vi "Stand Alone Init.vi"() -> (0 "error out":errorcluster, 1 "Engine Parent Editor Node":refnum<data-value>, 3 "Scan Engine Editor Node":refnum<data-value>)   [LabVIEW 2013, in "Scan Engine editor node.lvclass"]
uses:
  Scan Engine editor node.lvclass
  <vilib>/NI/Tag Bus Data Framework/Configuration Editor/Classes/Engine Parent/Engine Parent Editor Node.lvclass
  <vilib>/NI/Tag Bus/tag/tag descriptor.lvclass
  <vilib>/NI/Tag Bus/tag/Data Type.ctl
  module/configuration/Scan Engine configuration.lvclass
  <vilib>/NI/Module Execution Interface/Engine Configuration/engine configuration.lvclass
  <vilib>/NI/Tag Bus/tag/tag descriptor.lvclass/tag descriptor.ctl
  <vilib>/NI/Tag Bus/tag/write tag name.vi
  <vilib>/NI/Tag Bus/tag/write data type.vi
  <vilib>/NI/Tag Bus Data Framework/Configuration Editor/Classes/Engine Parent/write engine configuration.vi
panel:
  out "ignore":errorcluster
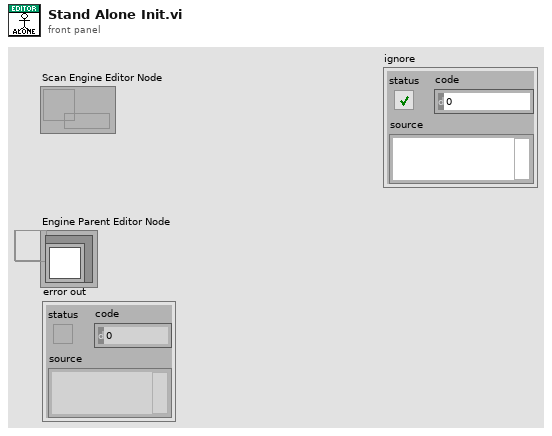
[diagram p1: front panel]
types:
  T1 = typedef "tag bus.lvlib/tag descriptor.lvclass/Data Type.ctl" = enum16{"Double", "Single", "I64", "I32", "I16", "I8", "U64", "U32", "U16", "U8", "Boolean", "String", "Array of Double", "Array of Single", "Array of I64", "Array of I32", "Array of I16", "Array of I8", "Array of U64", "Array of U32", "Array of U16", "Array of U8", "Array of Boolean", "Array of String"}
  T2 = typedef "NISE_CEF_Node.lvclass/NodeRef.ctl" = refnum<data-value>
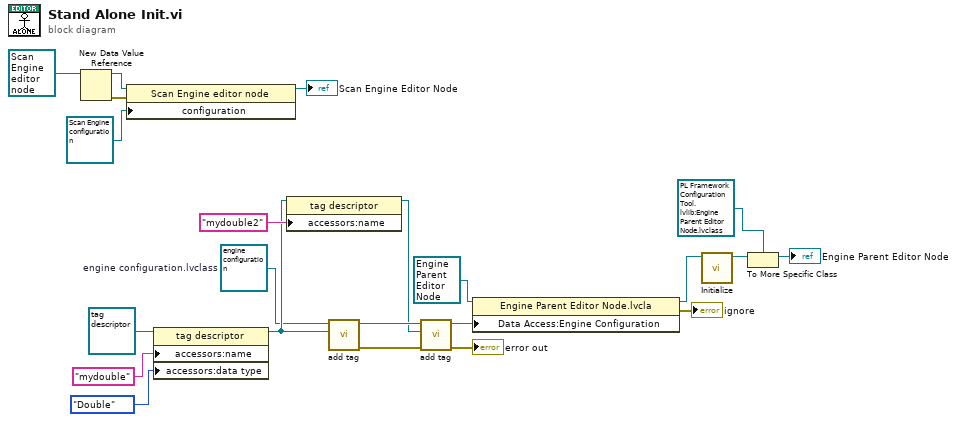
[diagram p0: block diagram]
diagram:
  w3 = refnum<class "engine configuration.lvclass"> refnum  # engine configuration.lvclass
  n1 = New Data Value Reference(data value=refnum<class "Scan Engine editor node.lvclass"> refnum ("Scan Engine editor node")) -> (data value reference=w10:refnum<data-value>, error out=w4:errorcluster)  [unwired: 1 in]
  n2 = property class="Scan Engine editor node"(reference=w10, error in=w4, "configuration"=refnum<class "Scan Engine configuration.lvclass"> refnum ("Scan Engine configuration")) -> (reference out=→"Scan Engine Editor Node":refnum<data-value>)  [unwired: 1 out]
  n3 = property class="tag descriptor"(reference=refnum<class "tag descriptor.lvclass"> refnum ("tag descriptor"), "accessors:name"="mydouble" ("name"), "accessors:data type"=Data_Type."Double" ("data type")) -> (reference out=w11:refnum<class "tag descriptor.lvclass">)  [unwired: 1 in, 1 out]
  n4 = property class="tag descriptor"(reference=w11, "accessors:name"="mydouble2" ("name")) -> (reference out=w12:refnum<class "tag descriptor.lvclass">)  [unwired: 1 in, 1 out]
  n5 = call <vilib>:"add tag.vi"("tag descriptor"=w11, "engine configuration in"=w3) -> ("error out"=w15:errorcluster, "engine configuration out"=w14:refnum<class "engine configuration.lvclass">)  [unwired: 8 in]
  n6 = call <vilib>:"add tag.vi"("error in"=w15, "tag descriptor"=w12, "engine configuration in"=w14) -> ("error out"=→"error out":errorcluster, "engine configuration out"=w1:refnum<class "engine configuration.lvclass">)  [unwired: 7 in]
  n7 = property class="Engine Parent Editor Node.lvcla"(reference=refnum<class "Engine Parent Editor Node.lvclass"> refnum ("PL Framework Configuration Tool.lvlib:Engine Parent Editor Node.lvclass"), "Data Access:Engine Configuration"=w1) -> (reference out=w6:refnum<class "Engine Parent Editor Node.lvclass">, error out=→"ignore":errorcluster)  [unwired: 1 in]
  n8 = call-dynamic "Initialize.vi"("Engine in"=w6) -> ("data value reference"=w22:T2)  [unwired: 8 in, 2 out]
  n9 = To More Specific Class(target class=refnum<data-value> refnum ("data value reference"), reference=w22) -> (specific class reference=→"Engine Parent Editor Node":refnum<data-value>)  [unwired: 1 in, 1 out]
